vi "FetchInputMessage.vi"(8 "error in (no error)":errorcluster, 11 "BaseDriver in":refnum<class "BaseDriver.lvclass">) -> (0 "error out":errorcluster, 3 "BaseDriver out":refnum<class "BaseDriver.lvclass">)   [LabVIEW 2013, in "BaseDriver.lvclass"]
doc: "Retrieves messages from the drivers input queue and parses them"
uses:
  BaseDriver.lvclass
  BaseDriver.lvclass/BaseDriver.ctl
  response.ctl
  driver_status.ctl
  Message/BaseMessage/BaseMessage.lvclass
  Responder/BaseResponder/BaseResponder.lvclass
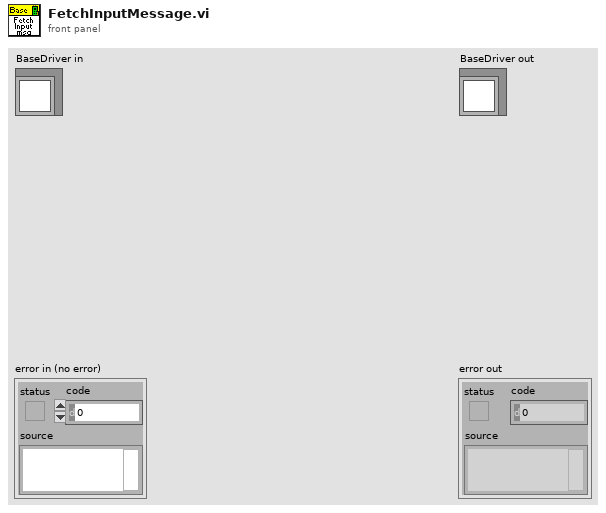
[diagram p1: front panel]
types:
  T1 = typedef "response.ctl" = cluster{"driver status":T2, "Sender":string, "Type":i32, "Variant":variant}
  T2 = typedef "driver_status.ctl" = enum16{"Normal", "Startup", "Connection lost", "Reconnected", "Timeout", "Idle", "Busy"}
  T3 = typedef "message_queue.ctl" = refnum<queue>
  T4 = typedef "driver_state.ctl" = enum16{"Idle", "Wait for ack"}
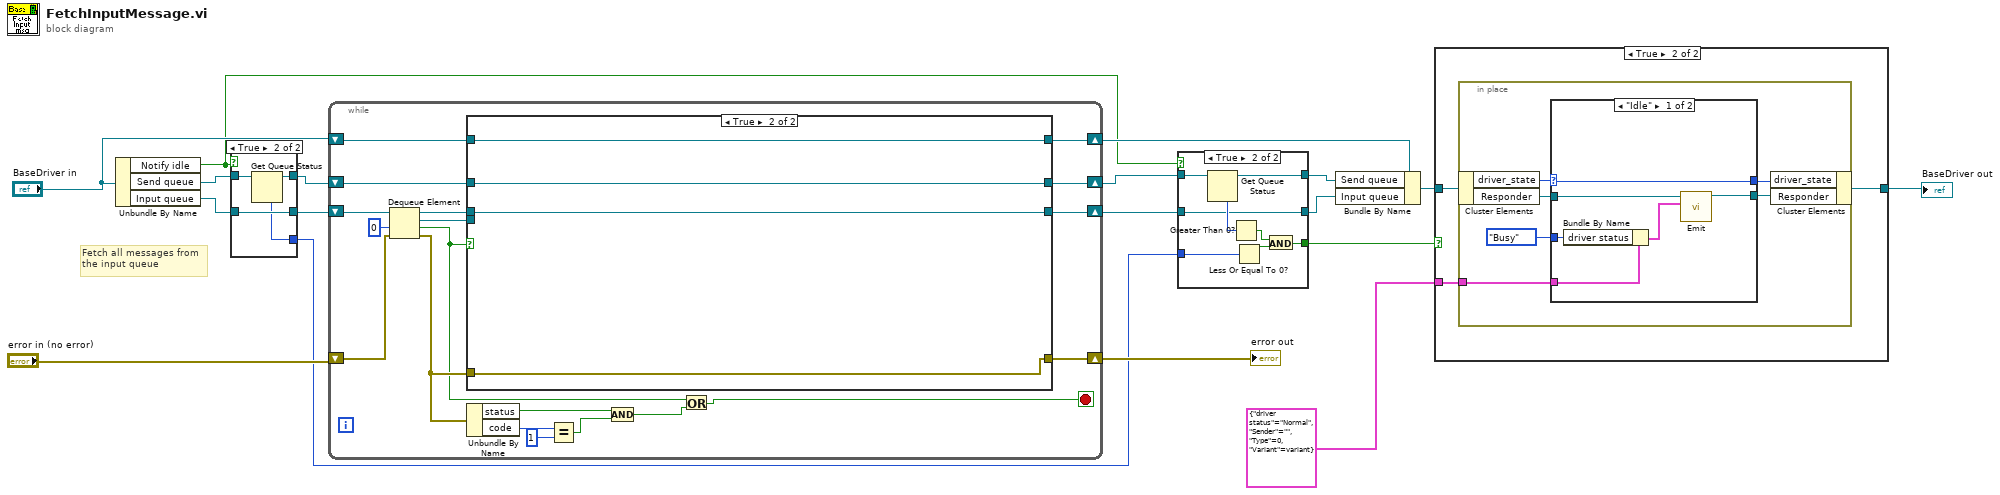
[diagram p0: block diagram]
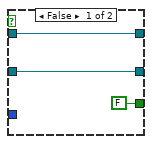
[diagram p2: hidden frame]
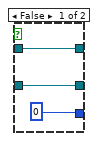
[diagram p3: hidden frame]
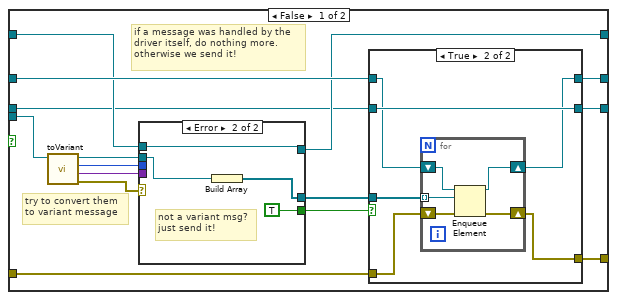
[diagram p6: hidden frame]
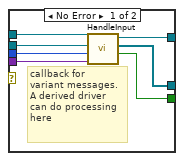
[diagram p8: hidden frame]
diagram:
  # "Fetch all messages from\nthe input queue"
  n1 = Unbundle By Name("BaseDriver in") -> ("Notify idle"=w3:bool, "Send queue"=w14:T3, "Input queue"=w6:T3)
  n2 = case shown="True" w3 {
    tunnel: w14 -> [w21 w25]
    tunnel: [w21 w24] -> w13
    tunnel: [0 ("# elements in queue") w22] -> w10
    tunnel: w6 -> [w20 w23]
    tunnel: [w20 w23] -> w5
    frame False {
    }
    frame True {
      n3 = Get Queue Status(queue=w25) -> (queue out=w24:T3, # elements in queue=w22:i32)  [unwired: 2 in, 6 out]
    }
  }
  n4 = while {
    shift-right: [w34] -> w1
    shift-left: w5 -> [w43]
    shift-right: [w41] -> w12
    shift-left: w13 -> [w42]
    shift-right: [w39] -> w17
    shift-left: "error in (no error)" -> [w40]
    shift-right: [w36] -> w15
    shift-left: "BaseDriver in" -> [w37]
    stop <- w26 stop-if-true
    n5 = Dequeue Element(queue=w43, timeout in ms (-1)=0, error in (no error)=w40) -> (queue out=w35:T3, element=w38:refnum<class "BaseMessage.lvclass">, timed out?=w28:bool, error out=w33:errorcluster)
    n6 = case shown="True" w28 {
      tunnel: w42 -> [w59 w87]
      tunnel: [w58 w87] -> w41
      tunnel: [w57 w85] -> w39
      tunnel: w38 -> [w56 _]
      tunnel: w37 -> [w51 w88]
      tunnel: [w50 w88] -> w36
      tunnel: w35 -> [w49 w86]
      tunnel: [w48 w86] -> w34
      tunnel: w33 -> [w46 w85]
      frame False {
        # "if a message was handled by the\ndriver itself, do nothing more.\notherwise we send it!"
        # "try to convert them\nto variant message"
        n7 = call-dynamic "toVariant.vi"("BaseMessage in"=w56) -> ("error out"=w55:errorcluster, "Variant"=w54:variant, "Type"=w53:i32, "BaseMessage out"=w52:refnum<class "BaseMessage.lvclass">)  [unwired: 7 in]
        n8 = case shown="Error" w55 {
          tunnel: w54 -> [w76 _]
          tunnel: w53 -> [w77 _]
          tunnel: w52 -> [w78 w82]
          tunnel: w51 -> [w80 w84]
          tunnel: [w79 w84] -> w50
          tunnel: [w75 w81] -> w47
          tunnel: [w74 TRUE ("Send message?")] -> w45
          frame No Error {
            # "callback for \nvariant messages.\nA derived driver\ncan do processing\nhere"
            n9 = call-dynamic "HandleInput.vi"("Variant"=w76, "Type"=w77, "Messge in"=w78, "BaseDriver in"=w80) -> ("Send message?"=w74:bool, "Messages out"=w75:refnum<class "BaseMessage.lvclass">[], "BaseDriver out"=w79:refnum<class "BaseDriver.lvclass">)  [unwired: 5 in]
          }
          frame Error {
            # "not a variant msg?\njust send it!"
            n10 = Build Array(w82) -> (w81:refnum<class "BaseMessage.lvclass">[])
          }
        }
        n11 = case shown="True" w45 {
          tunnel: w59 -> [w62 w66]
          tunnel: [w62 w65] -> w58
          tunnel: w46 -> [w60 w63]
          tunnel: [w60 w64] -> w57
          tunnel: w49 -> [w61 w68]
          tunnel: [w61 w68] -> w48
          tunnel: w47 -> [_ w67]
          frame False {
          }
          frame True {
            n12 = for {
              tunnel: w67 -> [w72] mode=indexing
              shift-right: [w70] -> w65
              shift-left: w66 -> [w71]
              shift-right: [w69] -> w64
              shift-left: w63 -> [w73]
              n13 = Enqueue Element(queue=w71, element=w72, error in (no error)=w73) -> (queue out=w70:T3, error out=w69:errorcluster)  [unwired: 1 in, 1 out]
            }
          }
        }
      }
      frame True {
      }
    }
    n14 = Unbundle By Name(w33) -> ("status"=w30:bool, "code"=w32:i32)
    n15 = Equal?(x=w32, y=1) -> (x = y?=w29:bool)
    n16 = And(x=w30, y=w29) -> (x .and. y?=w27:bool)
    n17 = Or(x=w28, y=w27) -> (x .or. y?=w26:bool)
  }
  "error out" <- w17
  n18 = case shown="True" w3 {
    tunnel: w12 -> [w91 w99]
    tunnel: [w91 w98] -> w11
    tunnel: w10 -> [_ w96]
    tunnel: [FALSE w93] -> w8
    tunnel: w1 -> [w90 w92]
    tunnel: [w90 w92] -> w4
    frame False {
    }
    frame True {
      n19 = Get Queue Status(queue=w99) -> (queue out=w98:T3, # elements in queue=w97:i32)  [unwired: 2 in, 6 out]
      n20 = Greater Than 0?(x=w97) -> (x > 0?=w95:bool)
      n21 = Less Or Equal To 0?(x=w96) -> (x <= 0?=w94:bool)
      n22 = And(x=w95, y=w94) -> (x .and. y?=w93:bool)
    }
  }
  n23 = Bundle By Name(cluster=w15, "Send queue"=w11, "Input queue"=w4) -> (w9:refnum<class "BaseDriver.lvclass">)
  n24 = case shown="True" w8 {
    tunnel: w9 -> [w100 w103]
    tunnel: T1 {"driver status"=enum."Normal", "Sender"="", "Type"=0, "Variant"=variant} ("response") -> [_ w101]
    tunnel: [w100 w102] -> w7
    frame False {
    }
    frame True {
      n25 = in-place "In Place Element Structure" {
        in-place-border: w101 -> [w104]
        n26 = in-place-cluster #1(w103) -> ("driver_state"=w106:T4, "Responder"=w109:refnum<class "BaseResponder.lvclass">)
        n27 = case shown="\"Idle\"" w106 {
          selector: w106 -> [w111 w117]
          tunnel: w109 -> [w115 w116]
          tunnel: [w114 w116] -> w108
          tunnel: w104 -> [w110 _]
          tunnel: driver_status."Busy" ("driver status") -> [w113 _]
          tunnel: [w111 w117] -> w105
          frame "Idle" {
            n28 = Bundle By Name(cluster=w110, "driver status"=w113) -> (w112:T1)
            n29 = call-dynamic "Emit.vi"("response"=w112, "BaseResponder in"=w115) -> ("BaseResponder out"=w114:refnum<class "BaseResponder.lvclass">)  [unwired: 8 in, 1 out]
          }
          frame "Wait for ack" {
          }
        }
        n30 = in-place-cluster #1("driver_state"=w105, "Responder"=w108) -> (w102:refnum<class "BaseDriver.lvclass">)
      }
    }
  }
  "BaseDriver out" <- w7
